vi "map-sparkle-manage.vi"(0 "icicle array IN":T2[](array[typedef]), 1 "action":T1, 5 "string array IN":string[](array[string]), 11 "string in":string) -> (4 "icicle array OUT":T2[](array[typedef]), 6 "string array OUT":string[](array[string]), 8 "number array out":dbl[](array[numeric]), 10 "number out":dbl, 15 "string out":string)   [LabVIEW 2020]
uses:
  icicle.ctl
  array-icicle-manage-action.ctl
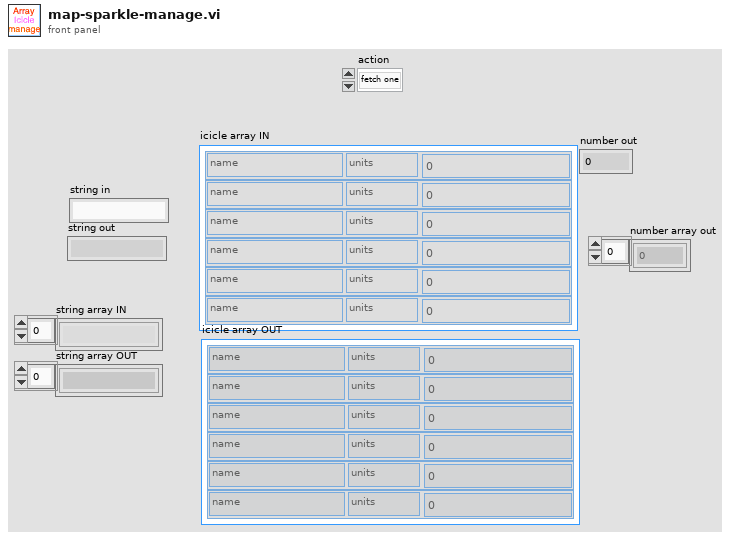
[diagram p1: front panel]
types:
  T1 = typedef "array-icicle-manage-action.ctl" = enum16{"fetch one", "fetch a few"}
  T2 = typedef "icicle.ctl" = cluster{"name":string, "units":string, "data":dbl}
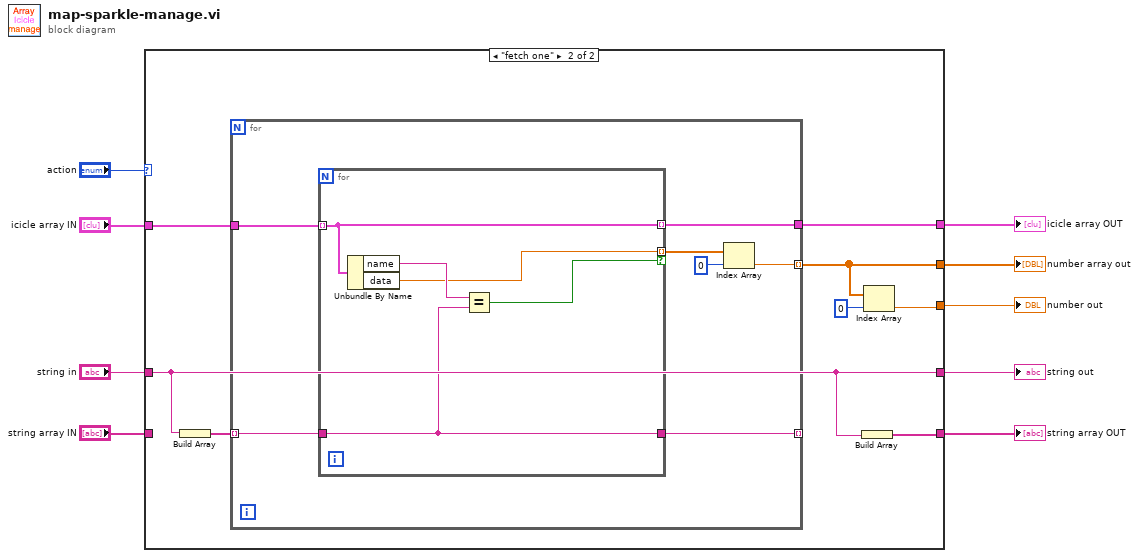
[diagram p0: block diagram]
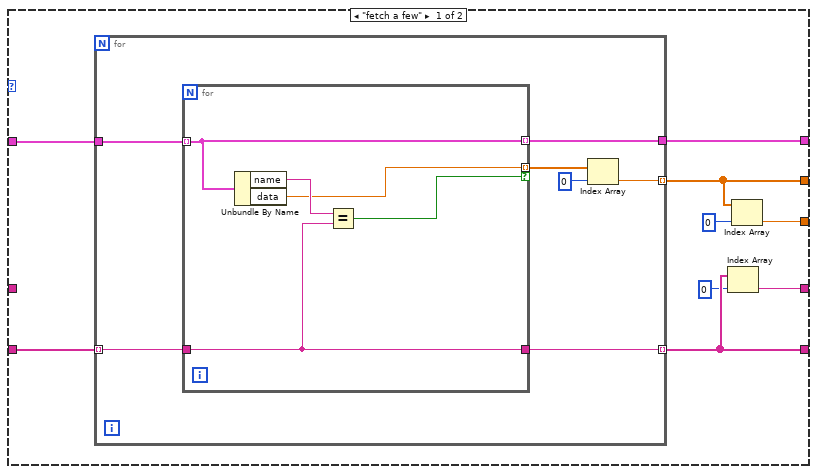
[diagram p2: hidden frame]
diagram:
  n1 = case shown="\"fetch one\"" "action" {
    tunnel: "icicle array IN" -> [w18 w38]
    tunnel: "string in" -> [_ w32]
    tunnel: [w17 w37] -> w6
    tunnel: [w13 w32] -> w5
    tunnel: [w14 w33] -> w4
    tunnel: "string array IN" -> [w16 _]
    tunnel: [w15 w34] -> w2
    tunnel: [w12 w31] -> w1
    frame "fetch a few" {
      n2 = for {
        tunnel: w18 -> [w25]
        tunnel: [w24] -> w17
        tunnel: w16 -> [w21] mode=indexing
        tunnel: [w20] -> w15 mode=indexing
        tunnel: [w19] -> w12 mode=indexing
        n3 = for {
          tunnel: w25 -> [w27] mode=indexing
          tunnel: [w29] -> w23 mode=indexing if=w28
          tunnel: [w27] -> w24 mode=indexing
          tunnel: [w26] -> w19
          tunnel: w21 -> [w26]
          n4 = Unbundle By Name(w27) -> ("name"=w30:string, "data"=w29:dbl)
          n5 = Equal?(x=w30, y=w26) -> (x = y?=w28:bool)
        }
        n6 = Index Array(array=w23, index=0) -> (element=w20:dbl)
      }
      n7 = Index Array(array=w12, index=0) -> (element=w13:string)
      n8 = Index Array(array=w15, index=0) -> (element=w14:dbl)
    }
    frame "fetch one" {
      n9 = Build Array(w32) -> (w36:string[])
      n10 = for {
        tunnel: w38 -> [w45]
        tunnel: [w44] -> w37
        tunnel: w36 -> [w41] mode=indexing
        tunnel: [w40] -> w34 mode=indexing
        tunnel: [w39] -> _ mode=indexing
        n11 = for {
          tunnel: w45 -> [w47] mode=indexing
          tunnel: [w49] -> w43 mode=indexing if=w48
          tunnel: [w47] -> w44 mode=indexing
          tunnel: [w46] -> w39
          tunnel: w41 -> [w46]
          n12 = Unbundle By Name(w47) -> ("name"=w50:string, "data"=w49:dbl)
          n13 = Equal?(x=w50, y=w46) -> (x = y?=w48:bool)
        }
        n14 = Index Array(array=w43, index=0) -> (element=w40:dbl)
      }
      n15 = Build Array(w32) -> (w31:string[])
      n16 = Index Array(array=w34, index=0) -> (element=w33:dbl)
    }
  }
  "icicle array OUT" <- w6
  "string out" <- w5
  "number out" <- w4
  "string array OUT" <- w1
  "number array out" <- w2
